vi "Configure Math.vi"(0 "VISA resource name":refnum<visa-resource-name>, 1 "Math Format (2: Percent)":u16(ring)=2 items=["None", "Linear Scaling and Offset", "Percent", "Reciprocal"], 3 "Percent Reference Method (0: Manual)":u16(ring) items=["Manual", "Acquire"], 4 "Percent Reference Value (1)":dbl=1.0, 5 "error in (no error)":errorcluster, 6 "Channel List (Empty)":string, 7 "Scalar (1)":dbl=1.0, 9 "Offset (0)":dbl, 11 "Units (X)":string="X") -> (14 "VISA resource name out":refnum<visa-resource-name>, 19 "error out":errorcluster)   [LabVIEW 2020, in "Keithley 27XX.lvlib"]
doc: "There are three built-in math calculations that are accessed from this VI: Linear Scaling and Offset (mX+B), percent, and reciprocal (1/X).\n\nThis VI allows you to configure attributes of each of these calculations, as well as determine which, if any, you want to use."
uses:
  Keithley 27XX.lvlib
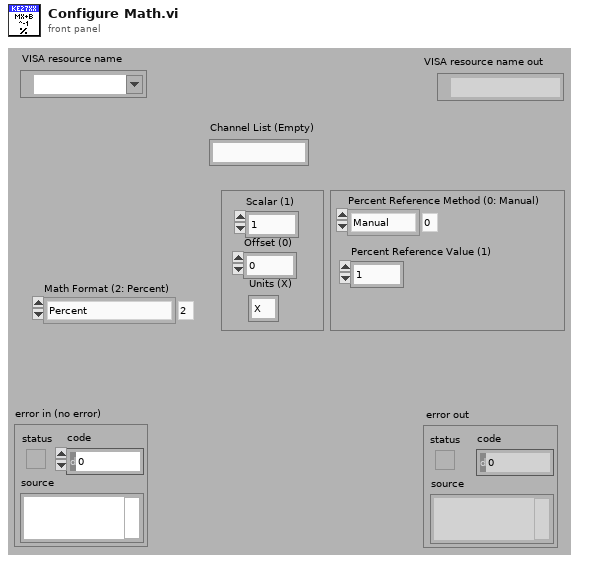
[diagram p1: front panel]
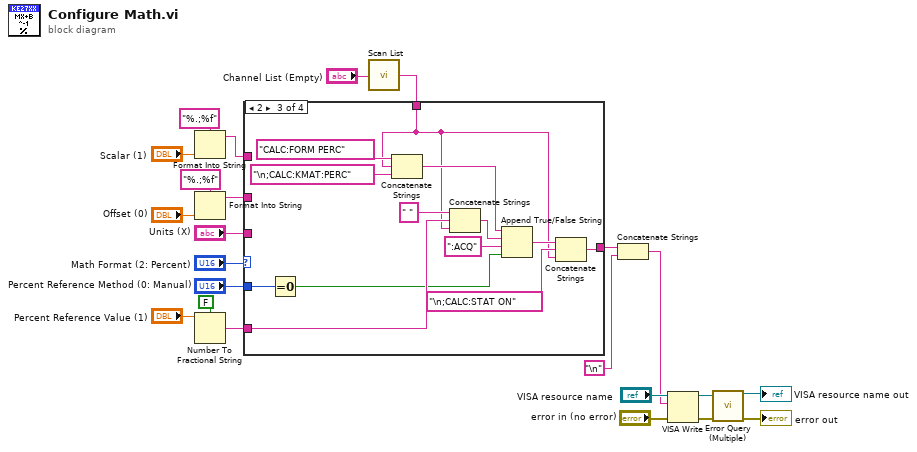
[diagram p0: block diagram]
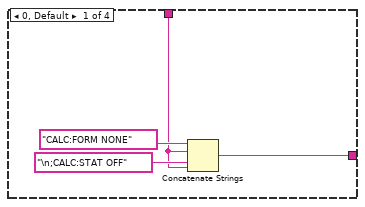
[diagram p2: hidden frame]
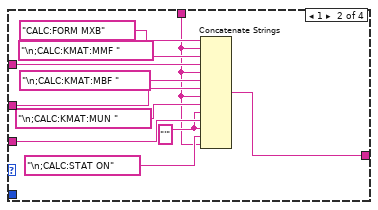
[diagram p3: hidden frame]
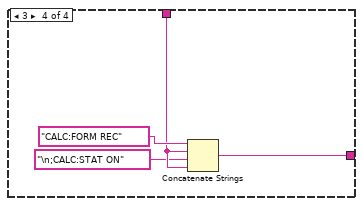
[diagram p4: hidden frame]
diagram:
  n1 = Format Into String(format string="%.;%f", "Scalar (1)") -> (resulting string=w14:string)  [unwired: 2 in, 1 out]
  n2 = Format Into String(format string="%.;%f", "Offset (0)") -> (resulting string=w12:string)  [unwired: 2 in, 1 out]
  n3 = Number To Fractional String(use system decimal point (T)=FALSE, number="Percent Reference Value (1)") -> (F-format string=w19:string)  [unwired: 2 in]
  n4 = call "Scan List.vi"("Scan List (Empty)"="Channel List (Empty)") -> ("Scan List Out"=w5:string)  [unwired: 14 in]
  n5 = case shown="2" "Math Format (2: Percent)" {
    tunnel: w5 -> [w24 w28 w39 w54]
    tunnel: w14 -> [_ w36 _ _]
    tunnel: w12 -> [_ w34 _ _]
    tunnel: "Units (X)" -> [_ w31 _ _]
    tunnel: "Percent Reference Method (0: Manual)" -> [_ _ w49 _]
    tunnel: w19 -> [_ _ w51 _]
    tunnel: [w26 w32 w41 w52] -> w4
    frame 0, Default {
      n6 = Concatenate Strings("CALC:FORM NONE", w24, "\n;CALC:STAT OFF" ("string (\"\")"), w24) -> (w26:string)
    }
    frame 1 {
      w30 = "'" ("string")
      n7 = Concatenate Strings("CALC:FORM MXB", w28, "\n;CALC:KMAT:MMF ", w36, w28, "\n;CALC:KMAT:MBF ", w34, w28, "\n;CALC:KMAT:MUN ", w30, w31, w30, "\n;CALC:STAT ON" ("string (\"\")"), w28) -> (w32:string)
    }
    frame 2 {
      n8 = Equal To 0?(x=w49) -> (x = 0?=w48:bool)
      n9 = Concatenate Strings("CALC:FORM PERC" ("string (\"\")"), w39, "\n;CALC:KMAT:PERC" ("string (\"\")")) -> (w43:string)
      n10 = Concatenate Strings(" " ("string (\"\")"), w51, w39) -> (w46:string)
      n11 = Append True/False String(1:w48, 2:":ACQ" ("false string"), 3:w46, 4:w43) -> (0:w42:string)
      n12 = Concatenate Strings(w42, "\n;CALC:STAT ON" ("string (\"\")"), w39) -> (w41:string)
    }
    frame 3 {
      n13 = Concatenate Strings("CALC:FORM REC", w54, "\n;CALC:STAT ON" ("string (\"\")"), w54) -> (w52:string)
    }
  }
  n14 = Concatenate Strings(w4, "\n") -> (w3:string)
  n15 = VISA Write(VISA resource name="VISA resource name", write buffer=w3, error in (no error)="error in (no error)") -> (VISA resource name out=w10:refnum<visa-resource-name>, error out=w9:errorcluster)  [unwired: 1 out]
  n16 = call "Error Query (Multiple).vi"("VISA resource name"=w10, "error in (no error)"=w9) -> ("VISA resource name out"=→"VISA resource name out":refnum<visa-resource-name>, "error out"=→"error out":errorcluster)  [unwired: 10 in, 2 out]
